vi "Set NumLock.vi"(8 "error in (no error)":errorcluster, 11 "Cursor in":refnum<class "Cursor.lvclass">) -> (0 "error out":errorcluster, 3 "Keypad out":refnum<class "Keypad.lvclass">)   [LabVIEW 2020, in "Keypad.lvlib" / "Cursor.lvclass"]
uses:
  Cursor.lvclass
  Numeric/Numeric.lvclass
  <vilib>/ni/Actors/State Actor/State Actor/State Actor.lvclass
  Keypad/Keypad.lvclass
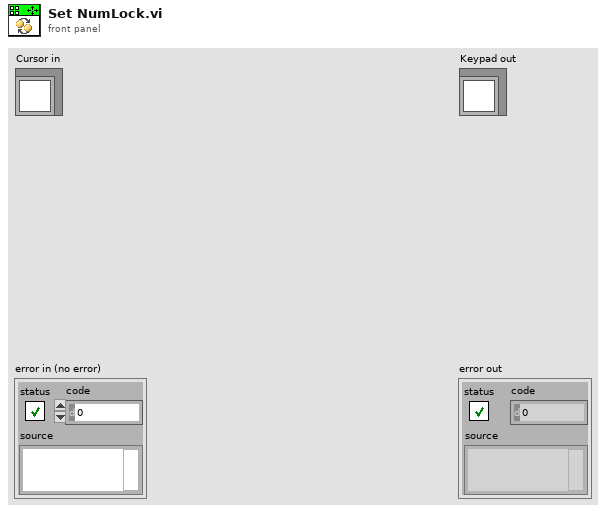
[diagram p1: front panel]
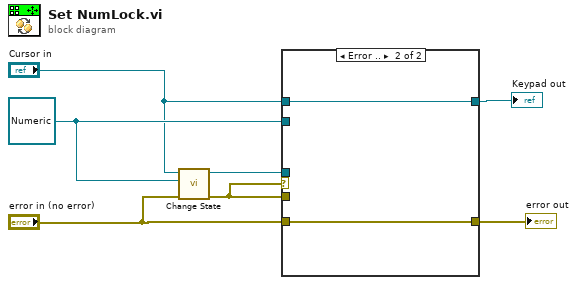
[diagram p0: block diagram]
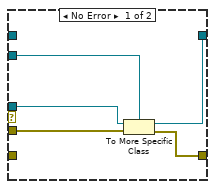
[diagram p2: hidden frame]
diagram:
  w6 = refnum<class "Numeric.lvclass"> refnum ("Keypad.lvlib:Numeric.lvclass")
  n1 = call <vilib>:"Change State.vi"("error in (no error)"="error in (no error)", "New State in"=w6, "State in"="Cursor in") -> ("error out"=w3:errorcluster, "State out"=w7:refnum<class "State Actor.lvclass">)  [unwired: 7 in]
  n2 = case shown="Error .." w3 {
    tunnel: w7 -> [w12 _]
    tunnel: w3 -> [w11 _]
    tunnel: w6 -> [w10 _]
    tunnel: [w9 w13] -> w5
    tunnel: [w8 w14] -> w4
    tunnel: "error in (no error)" -> [_ w14]
    tunnel: "Cursor in" -> [_ w13]
    frame No Error {
      n3 = To More Specific Class(target class=w10, reference=w12, error in=w11) -> (specific class reference=w9:refnum<class "Numeric.lvclass">, error out=w8:errorcluster)
    }
    frame Error {
    }
  }
  "error out" <- w4
  "Keypad out" <- w5
